vi "FPGA_ABEL_Kalman.vi"   [LabVIEW 2011]
uses:
  <vilib>/rvi/DataTransferAndStorage/Container/Common/niFpgaContainerState.ctl
  <vilib>/rvi/DataTransferAndStorage/Container/Common/niFpgaDataTypeControl.ctl
  <vilib>/rvi/DataTransferAndStorage/Container/Common/niFpgaContainerImplementationControl.ctl
  <vilib>/rvi/DataTransferAndStorage/Container/Common/niFpgaContainerArbitrationOptionsControl.ctl
  <vilib>/rvi/DataTransferAndStorage/Container/Common/niFpgaTransferTypeControl.ctl
  <vilib>/rvi/DataTransferAndStorage/Container/Common/niFpgaContainerInitializationParameters.ctl
  <vilib>/rvi/Memory/Memory_Types/niFpgaMemoryInterfaceConfiguration.ctl
  <vilib>/rvi/FIFO/Fifo_Types/niFpgaFifoControlLogicControl.ctl
  <vilib>/rvi/DataTransferAndStorage/Container/Common/niFpgaContainerMetaDataKey.ctl
  <vilib>/Platform/TimedLoop/XDataNode/timing_clust.ctl
  <vilib>/Platform/TimedLoop/XDataNode/nitl_modes.ctl
  <vilib>/Platform/TimedLoop/XDataNode/wakeup.ctl
  <vilib>/rvi/DataTransferAndStorage/Container/Common/niFpgaContainerGetUniqueNameForEmu.vi
  <vilib>/rvi/DataTransferAndStorage/Container/Common/niFpgaContainerSetEmuInfo.vi
  <vilib>/rvi/eio/common/nirviEmuReportErrorAndStop.vi
  <vilib>/rvi/FIFO/Fifo_Resource/nirvififoEmulationSetSize.vi
  Instance           3 24Saved   FPGA_ABEL_Kalman .vi
  FPGA_Global.vi
  <vilib>/rvi/interface/RandomDataEmulation/nirviRandomDataFPGAFIFO.vi
  <vilib>/rvi/interface/RandomDataEmulation/niFpgaRandomDataHandleErrors.vi
  Instance           2 24Saved   FPGA_ABEL_Kalman .vi
  <vilib>/rvi/Memory/Memory_Emulation/niFpgaMemoryEmulationValidateCache.vi
  <vilib>/rvi/Memory/Memory_Emulation/nirvimemoryEmulationManagerCache_InsertValue.vi
  <vilib>/Utility/error.llb/Clear Errors.vi
  <vilib>/rvi/Memory/Memory_Emulation/nirvimemoryEmulationManagerCache_GetValue.vi
  <vilib>/rvi/eio/common/nirviEmuTemplateMethod_errors.vi
  Instance           1 24Saved   FPGA_ABEL_Kalman .vi
  Instance           7 24Saved   FPGA_ABEL_Kalman .vi
  <vilib>/rvi/Memory/Memory_Emulation/nirvimemoryEmulationManagerCache_SetValue.vi
  <vilib>/rvi/LocalResourceManager/LocalResourceManager.xnode
  <vilib>/Platform/TimedLoop/XDataNode/XDataNode.xnode
  <vilib>/rvi/DataTransferAndStorage/Container/XNode/niFpgaContainer.xnode
  <vilib>/rvi/FIFO/Fifo_Resource/nirvififoEmulationRead.vi
  <vilib>/rvi/Arithmetic/AddSubMult/XNode/nirviSatArithmetic.xnode
  <vilib>/rvi/interface/RandomDataEmulation/nirviRandomDataFpgaReadWriteTemplate.vi
  <vilib>/eio/EIONode/EIONode.xnode
  <vilib>/rvi/Memory/Memory_Emulation/nirvimemoryEmulation.vi
  <vilib>/rvi/FIFO/Fifo_Resource/nirvififoEmulationWrite.vi
  <vilib>/Platform/TimedLoop/XDataNode/XDNodeRunTimeDep.lvlib
  <vilib>/rvi/occurrence/nirviOccurrence.lvlib
types:
  T1 = typedef "XDNodeRunTimeDep.lvlib/timing_clust.ctl" = cluster{"Expected End [f-1]":u64, "Actual End [f-1]":u64, "Finished Late? [f-1]":bool, "Expected End [i-1]":u64, "Actual End [i-1]":u64, "Finished Late? [i-1]":bool, "Expected Start [i]":u64, "Actual Start [i]":u64, "Expected Start [f]":u64, "Actual Start [f]":u64, "Source Name":string, "Structure Name":string, "Period":i64, "Deadline":i64, "Offset":i64, "Start":i64, "Priority":i32, "Timeout":i32, "Mode":T2, "Wakeup Reason":T3, "Error":errorcluster, "Source Type":string, "Secondary Source Type":string, "Global End Time":u64, "Global Start Time":u64, "Frame Duration":u64, "Iteration Duration":u64, "Assigned CPU":i32, "I/O Scan Engine Mode":u32}
  T2 = typedef "XDNodeRunTimeDep.lvlib/nitl_modes.ctl" = enum32{"No Change", "Process missed periods, maintain original phase", "Discard missed periods, maintain original phase", "Process missed periods, ignore original phase", "Discard missed periods, ignore original phase"}
  T3 = typedef "XDNodeRunTimeDep.lvlib/wakeup.ctl" = enum32{"Normal", "Aborted", "Asynchronous wakeup", "Timing source error", "Timed loop error", "Timeout"}
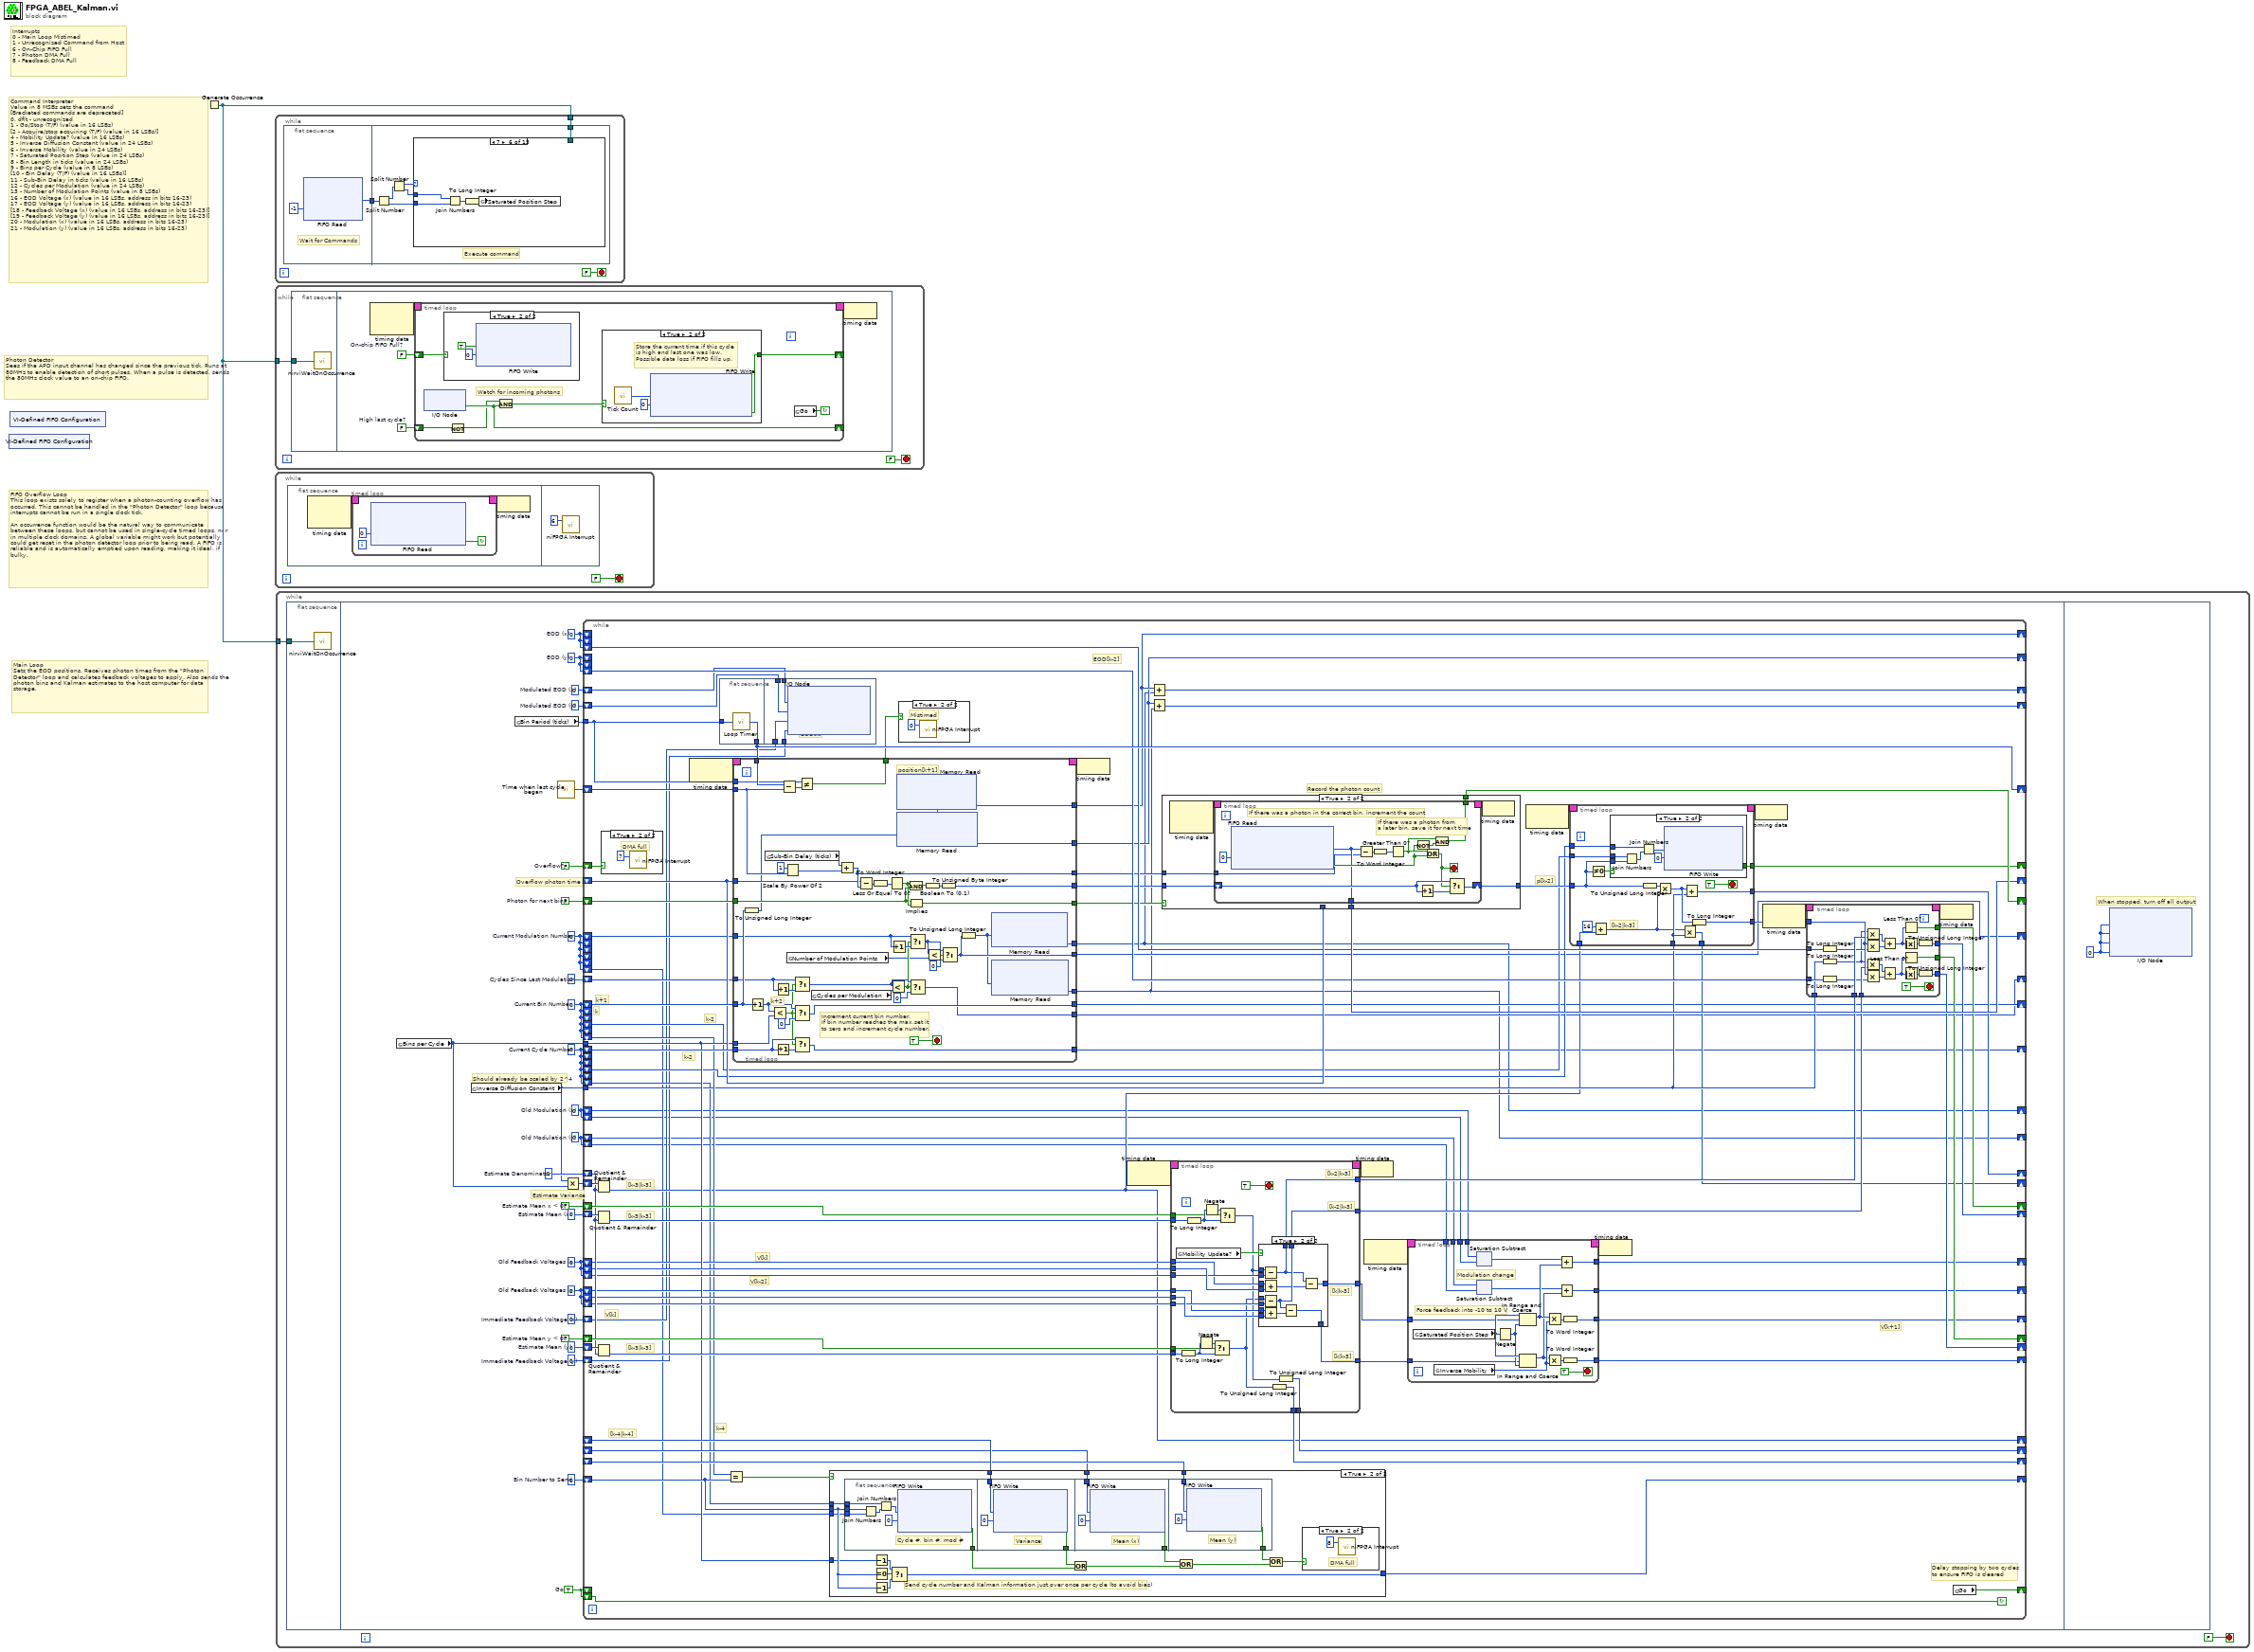
[diagram p0: block diagram]
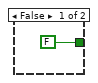
[diagram p3: hidden frame]
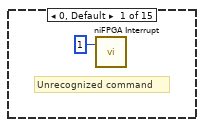
[diagram p4: hidden frame]
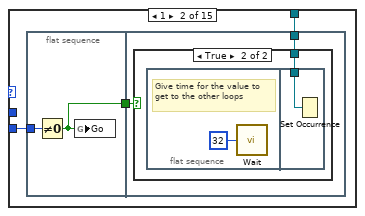
[diagram p5: hidden frame]
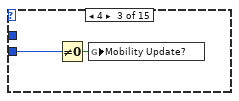
[diagram p7: hidden frame]
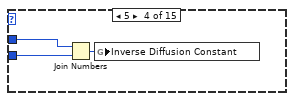
[diagram p8: hidden frame]
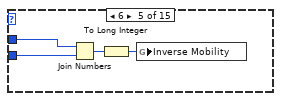
[diagram p9: hidden frame]
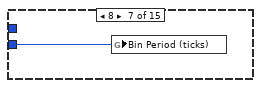
[diagram p10: hidden frame]
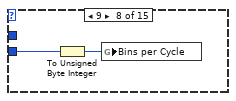
[diagram p11: hidden frame]
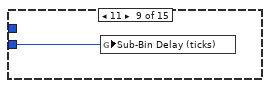
[diagram p12: hidden frame]
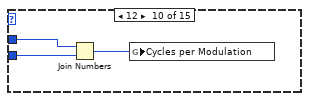
[diagram p13: hidden frame]
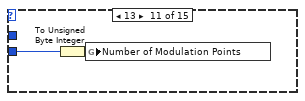
[diagram p14: hidden frame]
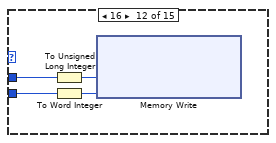
[diagram p15: hidden frame]
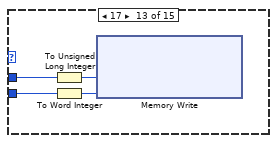
[diagram p16: hidden frame]
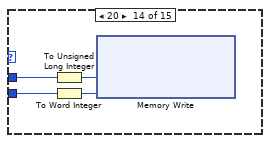
[diagram p17: hidden frame]
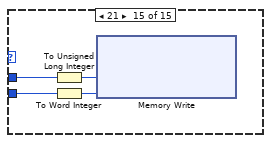
[diagram p18: hidden frame]
diagram:
  # "FIFO Overflow Loop\nThis loop exists solely to register when a photon-counting overflow has occurred. This cannot be handled in the \"Photon Detector\" loop because interrupts cannot be run in a single clock tick.\n\nAn occurrence function would be the natural way to communicate between these loops, but cannot be used in single-cycle timed loops, nor in multiple clock domains. A global variable might work but potentially could get reset in the photon detector loop prior to being read. A FIFO is reliable and is automatically emptied upon reading, making it ideal, if bulky."
  # "Interrupts\n0 - Main Loop Mistimed\n1 - Unrecognized Command from Host\n6 - On-Chip FIFO Full\n7 - Photon DMA Full\n8 - Feedback DMA Full"
  # "Command Interpreter\nValue in 8 MSBs sets the command\n[Bracketed commands are deprecated]\n0, dflt - unrecognized\n1 - Go/Stop (T/F) (value in 16 LSBs)\n[2 - Acquire/stop acquiring (T/F) (value in 16 LSBs)]\n4 - Mobility Update? (value in 16 LSBs)\n5 - Inverse Diffusion Constant (value in 24 LSBs)\n6 - Inverse Mobility (value in 24 LSBs)\n7 - Saturated Position Step (value in 24 LSBs)\n8 - Bin Length in ticks (value in 24 LSBs)\n9 - Bins per Cycle (value in 8 LSBs)\n[10 - Bin Delay (T/F) (value in 16 LSBs)]\n11 - Sub-Bin Delay in ticks (value in 16 LSBs)\n12 - Cycles per Modulation (value in 24 LSBs)\n13 - Number of Modulation Points (value in 8 LSBs)\n16 - EOD Voltage (x) (value in 16 LSBs, address in bits 16-23)\n17 - EOD Voltage (y) (value in 16 LSBs, address in bits 16-23)\n[18 - Feedback Voltage (x) (value in 16 LSBs, address in bits 16-23)]\n[19 - Feedback Voltage (y) (value in 16 LSBs, address in bits 16-23)]\n20 - Modulation (x) (value in 16 LSBs, address in bits 16-23)\n21 - Modulation (y) (value in 16 LSBs, address in bits 16-23)"
  # "Main Loop\nSets the EOD positions. Receives photon times from the \"Photon Detector\" loop and calculates feedback voltages to apply. Also sends the photon bins and Kalman estimates to the host computer for data storage."
  # "Photon Detector\nSees if the APD input channel has changed since the previous tick. Runs at 80MHz to enable detection of short pulses. When a pulse is detected, sends the 80MHz clock value to an on-chip FIFO."
  n1 = xnode "VI-Defined FIFO Configuration"() -> ()  [unwired: 1 out]
  n2 = xnode "VI-Defined FIFO Configuration"() -> ()  [unwired: 1 out]
  n3 = Generate Occurrence() -> (w1:refnum<k4>)
  n4 = while {
    tunnel: w1 -> [w2]
    stop <- FALSE stop-if-true
    n5 = flat-sequence {
      tunnel: [w5] -> w4
      tunnel: w4 -> [w12]
      tunnel: w2 -> [w7]
      frame #0 {
        # "Wait for Commands"
        n6 = xnode ("FIFO Read")("Timeout"=-1) -> ("Element"=w5:u32)  [unwired: 1 in, 2 out]
      }
      frame #1 {
        # "Execute command"
        n7 = Split Number(x=w12) -> (hi(x)=w11:u16, lo(x)=w8:u16)
        n8 = Split Number(x=w11) -> (hi(x)=w10:u8, lo(x)=w9:u8)
        n9 = case shown="7" w10 {
          tunnel: w9 -> [_ _ _ w27 w31 w35 _ _ _ w42 _ w49 w53 w57 w61]
          tunnel: w8 -> [_ w16 w25 w28 w32 w36 w37 w39 w40 w43 w45 w48 w52 w56 w60]
          tunnel: w7 -> [_ w15 _ _ _ _ _ _ _ _ _ _ _ _ _]
          frame 0, Default {
            # "Unrecognized command"
            n10 = call <vilib>:"niFPGA Interrupt.vi"("IRQ Number"=u8 1) -> ()  [unwired: 2 in]
          }
          frame 1 {
            n11 = flat-sequence {
              tunnel: w16 -> [w18]
              tunnel: [w17] -> w14
              tunnel: w15 -> [w20]
              tunnel: w14 -> [w19]
              frame #0 {
                n12 = Not Equal To 0?(x=w18) -> (x != 0?=w17:bool)
                n13 = global write "FPGA_Global.vi" "Go"(w17) -> ()
              }
              frame #1 {
                n14 = case shown="True" w19 {
                  tunnel: w20 -> [_ w21]
                  frame False {
                  }
                  frame True {
                    n15 = flat-sequence {
                      tunnel: w21 -> [w23]
                      frame #0 {
                        # "Give time for the value to get to the other loops"
                        n16 = call "Wait"("Count(Ticks)"=u8 32) -> ()  [unwired: 1 out]
                      }
                      frame #1 {
                        n17 = Set Occurrence(w23) -> ()
                      }
                    }
                  }
                }
              }
            }
          }
          frame 4 {
            n18 = Not Equal To 0?(x=w25) -> (x != 0?=w24:bool)
            n19 = global write "FPGA_Global.vi" "Mobility Update?"(w24) -> ()
          }
          frame 5 {
            n20 = Join Numbers(hi=w27, lo=w28) -> ((hi.lo)=w26:u32)
            n21 = global write "FPGA_Global.vi" "Inverse Diffusion Constant"(w26) -> ()
          }
          frame 6 {
            n22 = Join Numbers(hi=w31, lo=w32) -> ((hi.lo)=w30:u32)
            n23 = To Long Integer(number=w30) -> (32bit integer=w29:i32)
            n24 = global write "FPGA_Global.vi" "Inverse Mobility"(w29) -> ()
          }
          frame 7 {
            n25 = Join Numbers(hi=w35, lo=w36) -> ((hi.lo)=w34:u32)
            n26 = To Long Integer(number=w34) -> (32bit integer=w33:i32)
            n27 = global write "FPGA_Global.vi" "Saturated Position Step"(w33) -> ()
          }
          frame 8 {
            n28 = global write "FPGA_Global.vi" "Bin Period (ticks)"(w37) -> ()
          }
          frame 9 {
            n29 = To Unsigned Byte Integer(number=w39) -> (unsigned 8bit integer=w38:u8)
            n30 = global write "FPGA_Global.vi" "Bins per Cycle"(w38) -> ()
          }
          frame 11 {
            n31 = global write "FPGA_Global.vi" "Sub-Bin Delay (ticks)"(w40) -> ()
          }
          frame 12 {
            n32 = Join Numbers(hi=w42, lo=w43) -> ((hi.lo)=w41:u32)
            n33 = global write "FPGA_Global.vi" "Cycles per Modulation"(w41) -> ()
          }
          frame 13 {
            n34 = To Unsigned Byte Integer(number=w45) -> (unsigned 8bit integer=w44:u8)
            n35 = global write "FPGA_Global.vi" "Number of Modulation Points"(w44) -> ()
          }
          frame 16 {
            n36 = To Unsigned Long Integer(number=w49) -> (unsigned 32bit integer=w47:u32)
            n37 = To Word Integer(number=w48) -> (16bit integer=w46:i16)
            n38 = xnode ("Memory Write")("Address"=w47, "Data"=w46) -> ()  [unwired: 1 in, 1 out]
          }
          frame 17 {
            n39 = To Unsigned Long Integer(number=w53) -> (unsigned 32bit integer=w51:u32)
            n40 = To Word Integer(number=w52) -> (16bit integer=w50:i16)
            n41 = xnode ("Memory Write")("Address"=w51, "Data"=w50) -> ()  [unwired: 1 in, 1 out]
          }
          frame 20 {
            n42 = To Unsigned Long Integer(number=w57) -> (unsigned 32bit integer=w55:u32)
            n43 = To Word Integer(number=w56) -> (16bit integer=w54:i16)
            n44 = xnode ("Memory Write")("Address"=w55, "Data"=w54) -> ()  [unwired: 1 in, 1 out]
          }
          frame 21 {
            n45 = To Unsigned Long Integer(number=w61) -> (unsigned 32bit integer=w59:u32)
            n46 = To Word Integer(number=w60) -> (16bit integer=w58:i16)
            n47 = xnode ("Memory Write")("Address"=w59, "Data"=w58) -> ()  [unwired: 1 in, 1 out]
          }
        }
      }
    }
  }
  n48 = while {
    tunnel: w1 -> [w62]
    stop <- FALSE stop-if-true
    n49 = flat-sequence {
      tunnel: w62 -> [w64]
      frame #0 {
        n50 = call <vilib>:"nirviWaitOnOccurrence.vi"("occurrence"=w64) -> ()  [unwired: 4 in, 1 out]
      }
      frame #1 {
        w65 = FALSE  # On-chip FIFO Full?
        w66 = FALSE  # High last cycle?
        n51 = node-c288() -> (w68:T1)  [unwired: 2 in]
        n52 = timed-loop {
          timing: w68 -> [_]
          timing-out: [_] -> w67
          shift-right: [w71] -> _
          shift-left: w66 -> [w75]
          shift-right: [w72] -> _
          shift-left: w65 -> [w69]
          stop <- w73 continue-if-true
          # "Watch for incoming photons"
          n53 = xnode "I/O Node"() -> ("APD"=w71:bool)  [unwired: 1 in, 1 out]
          n54 = case shown="True" w69 {
            frame False {
            }
            frame True {
              n55 = xnode ("FIFO Write")("Element"=TRUE, "Timeout"=0) -> ()  [unwired: 2 in, 3 out]
            }
          }
          n56 = Not(x=w75) -> (.not. x?=w70:bool)
          n57 = And(x=w70, y=w71) -> (x .and. y?=w74:bool)
          n58 = case shown="True" w74 {
            tunnel: [FALSE ("Full") w79] -> w72
            frame False {
            }
            frame True {
              # "Store the current time if this cycle\nis high and last one was low.\nPossible data loss if FIFO fills up."
              n59 = call "Tick Count"() -> ("Tick Count(Ticks)"=w80:u16)
              n60 = xnode ("FIFO Write")("Element"=w80, "Timeout"=0) -> ("Timed Out?"=w79:bool)  [unwired: 1 in, 1 out]
            }
          }
          n61 = global read "FPGA_Global.vi" "Go"() -> (w73:bool)
        }
        n62 = node-c288(w67) -> ()
      }
    }
  }
  n63 = while {
    stop <- FALSE stop-if-true
    n64 = flat-sequence {
      frame #0 {
        n65 = node-c288() -> (w88:T1)  [unwired: 2 in]
        n66 = timed-loop {
          timing: w88 -> [_]
          timing-out: [_] -> w87
          stop <- w89 continue-if-true
          n67 = xnode ("FIFO Read")("Timeout"=0) -> ("Timed Out?"=w89:bool)  [unwired: 1 in, 2 out]
        }
        n68 = node-c288(w87) -> ()
      }
      frame #1 {
        n69 = call <vilib>:"niFPGA Interrupt.vi"("IRQ Number"=u8 6) -> ()  [unwired: 2 in]
      }
    }
  }
  n70 = while {
    tunnel: w1 -> [w96]
    stop <- FALSE stop-if-true
    n71 = flat-sequence {
      tunnel: w96 -> [w98]
      frame #0 {
        n72 = call <vilib>:"nirviWaitOnOccurrence.vi"("occurrence"=w98) -> ()  [unwired: 4 in, 1 out]
      }
      frame #1 {
        w100 = i16 0  # Old Modulation (y)
        w99 = i16 0  # Old Modulation (x)
        w102 = i16 0  # Modulated EOD (y)
        w103 = i16 0  # Modulated EOD (x)
        w101 = u8 0  # Current Modulation Number
        w104 = u32 0  # Cycles Since Last Modulation
        w110 = u8 0  # Bin Number to Send
        w111 = TRUE  # Go
        w108 = 0  # Old Feedback Voltages (y)
        w109 = 0  # Old Feedback Voltages (x)
        w112 = i16 0  # Immediate Feedback Voltage (y)
        w113 = i16 0  # Immediate Feedback Voltage (x)
        w118 = u32 1  # Estimate Denominator
        w120 = FALSE  # Estimate Mean y < 0?
        w121 = FALSE  # Estimate Mean x < 0?
        w122 = u32 0  # Estimate Mean (y)
        w123 = u32 0  # Estimate Mean (x)
        w124 = FALSE  # Overflow?
        w125 = FALSE  # Photon for next bin?
        w114 = i16 0  # EOD (y)
        w115 = i16 0  # EOD (x)
        w106 = u16 0  # Current Cycle Number
        w107 = u8 0  # Current Bin Number
        # "Should already be scaled by 2^4"
        # "Estimate Variance"
        # "Overflow photon time"
        n73 = global read "FPGA_Global.vi" "Bins per Cycle"() -> (w116:u8)
        n74 = global read "FPGA_Global.vi" "Inverse Diffusion Constant"() -> (w105:u32)
        n75 = global read "FPGA_Global.vi" "Bin Period (ticks)"() -> (w119:u16)
        n76 = call "Time when last cycle began"() -> ("Tick Count(Ticks)"=w126:u16)
        n77 = Multiply(x=w105, y=w116) -> (x*y=w117:u32)
        n78 = while {
          tunnel: w119 -> [w215]
          shift-right: [w139] -> _
          shift-left: w115 -> [_]
          shift-right: [w138] -> _
          shift-left: w114 -> [_]
          shift-right: [w147] -> _
          shift-left: w107 -> [w219]
          tunnel: w116 -> [w163]
          shift-right: [w148] -> _
          shift-left: w106 -> [w218]
          shift-left: w114 -> [_]
          shift-left: w115 -> [_]
          shift-right: [w216] -> _
          shift-left: w126 -> [w217]
          shift-right: [w214] -> _
          shift-left: w125 -> [w213]
          shift-right: [w212] -> _
          shift-left: _ -> [w211]
          shift-left: w106 -> [_]
          shift-left: w106 -> [_]
          shift-left: w107 -> [_]
          shift-left: w107 -> [_]
          shift-right: [w207] -> _
          shift-left: w124 -> [w206]
          shift-right: [w187] -> _
          shift-left: w123 -> [w200]
          shift-right: [w153] -> _
          shift-left: w117 -> [w201]
          tunnel: w105 -> [w156]
          shift-right: [w189] -> _
          shift-left: w122 -> [w198]
          shift-right: [w170] -> _
          shift-left: w113 -> [w141]
          shift-right: [w169] -> _
          shift-left: w112 -> [w140]
          shift-right: [w188] -> _
          shift-left: w120 -> [w202]
          shift-right: [w186] -> _
          shift-left: w121 -> [w203]
          shift-right: [w196] -> _
          shift-left: w118 -> [w181]
          shift-right: [w154] -> _
          shift-left: _ -> [w182]
          shift-right: [w195] -> _
          shift-left: _ -> [w179]
          shift-right: [w194] -> _
          shift-left: _ -> [w180]
          shift-left: w115 -> [w177]
          shift-left: w114 -> [w178]
          shift-right: [w167] -> _
          shift-left: w109 -> [w175]
          shift-left: w109 -> [w176]
          shift-right: [w168] -> _
          shift-left: w108 -> [w173]
          shift-left: w108 -> [w174]
          shift-right: [w166] -> _
          shift-left: w111 -> [_]
          shift-left: w111 -> [w165]
          shift-right: [w162] -> _
          shift-left: w110 -> [w164]
          shift-left: w107 -> [w161]
          shift-left: w107 -> [_]
          shift-left: w106 -> [w160]
          shift-left: w106 -> [_]
          shift-left: w109 -> [w159]
          shift-left: w108 -> [w158]
          shift-left: w107 -> [w157]
          shift-left: w106 -> [w155]
          shift-right: [w142] -> _
          shift-left: w104 -> [w150]
          shift-right: [w143] -> _
          shift-left: w101 -> [w149]
          shift-right: [w135] -> _
          shift-left: w103 -> [w137]
          shift-right: [w134] -> _
          shift-left: w102 -> [w136]
          shift-left: w101 -> [_]
          shift-left: w101 -> [_]
          shift-left: w101 -> [_]
          shift-left: w101 -> [_]
          shift-left: w101 -> [w133]
          shift-right: [w130] -> _
          shift-left: w99 -> [w131]
          shift-right: [w129] -> _
          shift-left: w100 -> [w128]
          shift-left: w99 -> [w132]
          shift-left: w100 -> [w127]
          stop <- w165 continue-if-true
          # "V[k-2]"
          # "V[k]"
          # "EOD[k-2]"
          # "k-2"
          # "k-4"
          # "Delay stopping by two cycles\nto ensure FIFO is cleared"
          # "V[k]"
          # "[k-3|k-3]"
          # "[k-3|k-3]"
          # "[k-4|k-4]"
          # "[k-3|k-3]"
          # "k-2"
          # "k"
          # "k+1"
          # "p[k-2]"
          # "V[k+1]"
          # "Record the photon count"
          n79 = Quotient & Remainder(x=w201, y=w181) -> (floor(x/y)=w154:u32)  [unwired: 1 out]
          n80 = Quotient & Remainder(x=w200, y=w181) -> (floor(x/y)=w199:u32)  [unwired: 1 out]
          n81 = Quotient & Remainder(x=w198, y=w181) -> (floor(x/y)=w197:u32)  [unwired: 1 out]
          n82 = case shown="True" w206 {
            frame False {
            }
            frame True {
              # "DMA full"
              n83 = call <vilib>:"niFPGA Interrupt.vi"("IRQ Number"=u8 7) -> ()  [unwired: 2 in]
            }
          }
          n84 = node-c288() -> (w221:T1)  [unwired: 1 in]
          n85 = flat-sequence {
            tunnel: w215 -> [w497]
            tunnel: [w496] -> w216
            tunnel: w141 -> [w501]
            tunnel: w140 -> [w500]
            tunnel: w137 -> [w499]
            tunnel: w136 -> [w498]
            frame #0 {
              n86 = call "Loop Timer"("Count(Ticks)"=w497) -> ("Tick Count(Ticks)"=w496:u16)
            }
            frame #1 {
              # "EOD[k]"
              n87 = xnode ("I/O Node")("EODDriver(x)"=w499, "EODDriver(y)"=w498, "FeedbackVoltage (x)"=w501, "FeedbackVoltage(y)"=w500) -> ()  [unwired: 4 in, 4 out]
            }
          }
          n88 = Equal?(x=w157, y=w164) -> (x = y?=w193:bool)
          n89 = timed-loop {
            timing: w221 -> [_]
            timing-out: [_] -> w220
            tunnel: w219 -> [w487]
            tunnel: [w490] -> w139
            tunnel: [w489] -> w138
            tunnel: w163 -> [w486]
            tunnel: [w485] -> w147
            tunnel: w218 -> [w482]
            tunnel: [w481] -> w148
            tunnel: w216 -> [w480]
            tunnel: w217 -> [w477]
            tunnel: w215 -> [w478]
            tunnel: [w466] -> w146
            tunnel: w213 -> [w469]
            tunnel: [w468] -> w145
            tunnel: [w467] -> w144
            tunnel: w211 -> [w465]
            tunnel: [w464] -> w210
            tunnel: w150 -> [w459]
            tunnel: w149 -> [w455]
            tunnel: [w450] -> w143
            tunnel: [w448] -> w142
            tunnel: [w447] -> w130
            tunnel: [w446] -> w129
            stop <- TRUE stop-if-true
            # "k+2"
            # "position[k+1]"
            # "Increment current bin number.\nIf bin number reaches the max,set it\nto zero and increment cycle number."
            n90 = To Unsigned Long Integer(number=w487) -> (unsigned 32bit integer=w463:u32)
            n91 = Increment(x=w487) -> (x+1=w488:u8)
            n92 = global read "FPGA_Global.vi" "Sub-Bin Delay (ticks)"() -> (w462:u16)
            n93 = Less?(x=w488, y=w486) -> (x < y?=w460:bool)
            n94 = Increment(x=w459) -> (x+1=w461:u32)
            n95 = Increment(x=w482) -> (x+1=w483:u16)
            n96 = Subtract(x=w480, y=w477) -> (x-y=w479:u16)
            n97 = Scale By Power Of 2(n=1, x=w477) -> (x*2^n=w475:u16)
            n98 = global read "FPGA_Global.vi" "Number of Modulation Points"() -> (w445:u8)
            n99 = Select(t=w459, s=w460, f=w461) -> (s? t:f=w458:u32)
            n100 = Select(t=w488, s=w460, f=u8 0 ("Current Bin Number")) -> (s? t:f=w485:u8)
            n101 = Select(t=w482, s=w460, f=w483) -> (s? t:f=w481:u16)
            n102 = Not Equal?(x=w478, y=w479) -> (x != y?=w464:bool)
            n103 = global read "FPGA_Global.vi" "Cycles per Modulation"() -> (w444:u32)
            n104 = Add(x=w462, y=w475) -> (x+y=w466:u16)
            n105 = Subtract(x=w465, y=w466) -> (x-y=w471:u16)
            n106 = To Word Integer(number=w471) -> (16bit integer=w472:i16)
            n107 = Less Or Equal To 0?(x=w472) -> (x <= 0?=w470:bool)
            n108 = Less?(x=w458, y=w444) -> (x < y?=w454:bool)
            n109 = Increment(x=w455) -> (x+1=w456:u8)
            n110 = xnode ("Memory Read")("Address"=w463) -> ("Data"=w490:i16)  [unwired: 1 in, 1 out]
            n111 = xnode ("Memory Read")("Address"=w463) -> ("Data"=w489:i16)  [unwired: 1 in, 1 out]
            n112 = And(x=w470, y=w469) -> (x .and. y?=w474:bool)
            n113 = Implies(1:w470, 2:w469) -> (0:w467:bool)
            n114 = Select(t=w455, s=w454, f=w456) -> (s? t:f=w451:u8)
            n115 = Select(t=w458, s=w454, f=u32 0) -> (s? t:f=w448:u32)
            n116 = Boolean To (0,1)(Boolean=w474) -> (0, 1=w473:i16)
            n117 = Less?(x=w451, y=w445) -> (x < y?=w453:bool)
            n118 = To Unsigned Byte Integer(number=w473) -> (unsigned 8bit integer=w468:u8)
            n119 = Select(t=w451, s=w453, f=u8 0) -> (s? t:f=w450:u8)
            n120 = To Unsigned Long Integer(number=w450) -> (unsigned 32bit integer=w449:u32)
            n121 = xnode ("Memory Read")("Address"=w449) -> ("Data"=w447:i16)  [unwired: 1 in, 1 out]
            n122 = xnode ("Memory Read")("Address"=w449) -> ("Data"=w446:i16)  [unwired: 1 in, 1 out]
          }
          n123 = case shown="True" w193 {
            tunnel: w179 -> [_ w326]
            tunnel: w182 -> [_ w325]
            tunnel: w155 -> [_ w324]
            tunnel: w180 -> [_ w320]
            tunnel: w164 -> [w308 w315]
            tunnel: w163 -> [_ w311]
            tunnel: [w308 w312] -> w162
            tunnel: w133 -> [_ w309]
            frame False {
            }
            frame True {
              # "Send cycle number and Kalman information just over once per cycle (to avoid bias)"
              n124 = flat-sequence {
                tunnel: w324 -> [w332]
                tunnel: [w333] -> w323
                tunnel: w315 -> [w329]
                tunnel: w309 -> [w328]
                tunnel: [w335] -> w322
                tunnel: w325 -> [w336]
                tunnel: w326 -> [w339]
                tunnel: [w338] -> w321
                tunnel: [w341] -> w318
                tunnel: w320 -> [w342]
                frame #0 {
                  # "Cycle #, bin #, mod #"
                  n125 = Join Numbers(hi=w329, lo=w328) -> ((hi.lo)=w330:u16)
                  n126 = Join Numbers(hi=w332, lo=w330) -> ((hi.lo)=w331:u32)
                  n127 = xnode ("FIFO Write")("Element"=w331, "Timeout"=0) -> ("Timed Out?"=w333:bool)  [unwired: 1 in, 1 out]
                }
                frame #1 {
                  # "Variance"
                  n128 = xnode ("FIFO Write")("Element"=w336, "Timeout"=0) -> ("Timed Out?"=w335:bool)  [unwired: 1 in, 1 out]
                }
                frame #2 {
                  # "Mean (x)"
                  n129 = xnode ("FIFO Write")("Element"=w339, "Timeout"=0) -> ("Timed Out?"=w338:bool)  [unwired: 1 in, 1 out]
                }
                frame #3 {
                  # "Mean (y)"
                  n130 = xnode ("FIFO Write")("Element"=w342, "Timeout"=0) -> ("Timed Out?"=w341:bool)  [unwired: 1 in, 1 out]
                }
              }
              n131 = Decrement(x=w311) -> (x-1=w310:u8)
              n132 = Equal To 0?(x=w315) -> (x = 0?=w314:bool)
              n133 = Decrement(x=w315) -> (x-1=w313:u8)
              n134 = Select(t=w310, s=w314, f=w313) -> (s? t:f=w312:u8)
              n135 = Or(x=w322, y=w323) -> (x .or. y?=w317:bool)
              n136 = Or(x=w321, y=w317) -> (x .or. y?=w319:bool)
              n137 = Or(x=w318, y=w319) -> (x .or. y?=w316:bool)
              n138 = case shown="True" w316 {
                frame False {
                }
                frame True {
                  # "DMA full"
                  n139 = call <vilib>:"niFPGA Interrupt.vi"("IRQ Number"=u8 8) -> ()  [unwired: 2 in]
                }
              }
            }
          }
          n140 = case shown="True" w210 {
            frame False {
            }
            frame True {
              # "Mistimed"
              n141 = call <vilib>:"niFPGA Interrupt.vi"("IRQ Number"=u8 0) -> ()  [unwired: 2 in]
            }
          }
          n142 = node-c288(w220) -> ()
          n143 = node-c288() -> (w205:T1)  [unwired: 1 in]
          n144 = Add(x=w139, y=w130) -> (x+y=w135:i16)
          n145 = Add(x=w138, y=w129) -> (x+y=w134:i16)
          n146 = case shown="True" w144 {
            tunnel: w146 -> [_ w424]
            tunnel: [u8 0 w423] -> w192
            tunnel: [TRUE w422] -> w214
            tunnel: w145 -> [_ w421]
            tunnel: [w418 w420] -> w212
            tunnel: w211 -> [w418 _]
            frame False {
              # "Still not time to use the photon from last cycle!"
            }
            frame True {
              n147 = node-c288() -> (w426:T1)  [unwired: 2 in]
              n148 = timed-loop {
                timing: w426 -> [_]
                timing-out: [_] -> w425
                tunnel: w424 -> [w429]
                shift-right: [w438] -> w423
                shift-left: w421 -> [w436]
                tunnel: [w433] -> w422
                tunnel: [w430] -> w420
                stop <- w435 stop-if-true
                # "If there was a photon in the correct bin, increment the count"
                # "If there was a photon from\na later bin, save it for next time"
                n149 = xnode ("FIFO Read")("Timeout"=0) -> ("Element"=w430:u16, "Timed Out?"=w432:bool)  [unwired: 1 in, 1 out]
                n150 = Subtract(x=w430, y=w429) -> (x-y=w428:u16)
                n151 = To Word Integer(number=w428) -> (16bit integer=w427:i16)
                n152 = Greater Than 0?(x=w427) -> (x > 0?=w434:bool)
                n153 = Not(x=w432) -> (.not. x?=w431:bool)
                n154 = Increment(x=w436) -> (x+1=w437:u8)
                n155 = Or(x=w434, y=w432) -> (x .or. y?=w435:bool)
                n156 = And(x=w434, y=w431) -> (x .and. y?=w433:bool)
                n157 = Select(t=w436, s=w435, f=w437) -> (s? t:f=w438:u8)
              }
              n158 = node-c288(w425) -> ()
            }
          }
          n159 = timed-loop {
            timing: w205 -> [_]
            timing-out: [_] -> w204
            tunnel: w197 -> [w366]
            tunnel: w199 -> [w365]
            tunnel: [w346] -> w184
            tunnel: [w347] -> w183
            tunnel: w176 -> [w352]
            tunnel: w174 -> [w350]
            tunnel: w203 -> [w362]
            tunnel: w202 -> [w359]
            tunnel: [w358] -> w195
            tunnel: [w357] -> w194
            tunnel: w173 -> [w351]
            tunnel: [w356] -> w151
            tunnel: w175 -> [w353]
            tunnel: [w355] -> w152
            tunnel: w159 -> [w349]
            tunnel: w158 -> [w348]
            stop <- TRUE stop-if-true
            # "[k-2|k-3]"
            # "[k|k-3]"
            # "[k|k-3]"
            # "[k-2|k-3]"
            n160 = global read "FPGA_Global.vi" "Mobility Update?"() -> (w354:bool)
            n161 = To Long Integer(number=w366) -> (32bit integer=w360:i32)
            n162 = To Long Integer(number=w365) -> (32bit integer=w363:i32)
            n163 = Negate(x=w360) -> (-x=w361:i32)
            n164 = Negate(x=w363) -> (-x=w364:i32)
            n165 = Select(t=w361, s=w359, f=w360) -> (s? t:f=w344:i32)
            n166 = Select(t=w364, s=w362, f=w363) -> (s? t:f=w345:i32)
            n167 = case shown="True" w354 {
              tunnel: w350 -> [_ w383]
              tunnel: w352 -> [_ w382]
              tunnel: w345 -> [w369 w381]
              tunnel: w344 -> [w368 w380]
              tunnel: w351 -> [_ w371]
              tunnel: [w368 w379] -> w347
              tunnel: [w368 w378] -> w356
              tunnel: w353 -> [_ w375]
              tunnel: [w369 w377] -> w346
              tunnel: [w369 w376] -> w355
              tunnel: w349 -> [_ w374]
              tunnel: w348 -> [_ w370]
              frame False {
              }
              frame True {
                n168 = Subtract(x=w381, y=w382) -> (x-y=w377:i32)
                n169 = Add(x=w374, y=w375) -> (x+y=w373:i32)
                n170 = Subtract(x=w380, y=w383) -> (x-y=w379:i32)
                n171 = Add(x=w370, y=w371) -> (x+y=w372:i32)
                n172 = Subtract(x=w379, y=w372) -> (x-y=w378:i32)
                n173 = Subtract(x=w377, y=w373) -> (x-y=w376:i32)
              }
            }
            n174 = To Unsigned Long Integer(number=w344) -> (unsigned 32bit integer=w357:u32)
            n175 = To Unsigned Long Integer(number=w345) -> (unsigned 32bit integer=w358:u32)
          }
          n176 = node-c288(w204) -> ()
          n177 = node-c288() -> (w172:T1)  [unwired: 1 in]
          n178 = timed-loop {
            timing: w172 -> [_]
            timing-out: [_] -> w171
            tunnel: [w236] -> w170
            tunnel: [w235] -> w169
            tunnel: [w224] -> w168
            tunnel: [w228] -> w167
            tunnel: w151 -> [w234]
            tunnel: w152 -> [w233]
            tunnel: w132 -> [w231]
            tunnel: w131 -> [w230]
            tunnel: w128 -> [w226]
            tunnel: w127 -> [w225]
            stop <- TRUE stop-if-true
            # "Modulation change"
            # "Force feedback into -10 to 10 V"
            n179 = global read "FPGA_Global.vi" "Saturated Position Step"() -> (w238:i32)
            n180 = global read "FPGA_Global.vi" "Inverse Mobility"() -> (w240:i32)
            n181 = xnode "Saturation Subtract"("x"=w230, "y"=w231) -> ("x-y"=w222:i32)
            n182 = xnode "Saturation Subtract"("x"=w226, "y"=w225) -> ("x-y"=w223:i32)
            n183 = Negate(x=w238) -> (-x=w237:i32)
            n184 = In Range and Coerce(upper limit=w238, x=w233, lower limit=w237) -> (coerced(x)=w229:i32)  [unwired: 1 out]
            n185 = In Range and Coerce(upper limit=w238, x=w234, lower limit=w237) -> (coerced(x)=w227:i32)  [unwired: 1 out]
            n186 = Multiply(x=w229, y=w240) -> (x*y=w239:i32)
            n187 = Multiply(x=w227, y=w240) -> (x*y=w241:i32)
            n188 = Add(x=w222, y=w229) -> (x+y=w228:i32)
            n189 = Add(x=w223, y=w227) -> (x+y=w224:i32)
            n190 = To Word Integer(number=w239) -> (16bit integer=w236:i16)
            n191 = To Word Integer(number=w241) -> (16bit integer=w235:i16)
          }
          n192 = node-c288() -> (w209:T1)  [unwired: 1 in]
          n193 = timed-loop {
            timing: w209 -> [_]
            timing-out: [_] -> w208
            tunnel: w192 -> [w397]
            tunnel: w160 -> [w401]
            tunnel: w161 -> [w400]
            tunnel: [w399] -> w207
            tunnel: w156 -> [w393]
            tunnel: [w394] -> w196
            tunnel: [w395] -> w185
            tunnel: w154 -> [w391]
            tunnel: [w392] -> w153
            stop <- TRUE stop-if-true
            # "[k-2|k-3]"
            n194 = Not Equal To 0?(x=w397) -> (x != 0?=w402:bool)
            n195 = Add(x=u32 16, y=w391) -> (x+y=w390:u32)
            n196 = case shown="True" w402 {
              tunnel: w397 -> [_ w410]
              tunnel: w401 -> [_ w409]
              tunnel: w400 -> [_ w408]
              tunnel: [FALSE ("Full") w405] -> w399
              frame False {
              }
              frame True {
                n197 = Join Numbers(hi=w408, lo=w410) -> ((hi.lo)=w411:u16)
                n198 = Join Numbers(hi=w409, lo=w411) -> ((hi.lo)=w407:u32)
                n199 = xnode ("FIFO Write")("Element"=w407, "Timeout"=0) -> ("Timed Out?"=w405:bool)  [unwired: 1 in, 1 out]
              }
            }
            n200 = To Unsigned Long Integer(number=w397) -> (unsigned 32bit integer=w398:u32)
            n201 = Multiply(x=w398, y=w390) -> (x*y=w396:u32)
            n202 = Multiply(x=w390, y=w393) -> (x*y=w392:u32)
            n203 = Add(x=w396, y=w393) -> (x+y=w394:u32)
            n204 = To Long Integer(number=w396) -> (32bit integer=w395:i32)
          }
          n205 = node-c288(w171) -> ()
          n206 = node-c288(w208) -> ()
          n207 = node-c288() -> (w191:T1)  [unwired: 1 in]
          n208 = timed-loop {
            timing: w191 -> [_]
            timing-out: [_] -> w190
            tunnel: [w299] -> w189
            tunnel: [w298] -> w188
            tunnel: [w297] -> w187
            tunnel: [w296] -> w186
            tunnel: w185 -> [w293]
            tunnel: w177 -> [w287]
            tunnel: w178 -> [w284]
            tunnel: w156 -> [w283]
            tunnel: w184 -> [w290]
            tunnel: w183 -> [w289]
            stop <- TRUE stop-if-true
            n209 = To Long Integer(number=w287) -> (32bit integer=w286:i32)
            n210 = To Long Integer(number=w283) -> (32bit integer=w282:i32)
            n211 = To Long Integer(number=w284) -> (32bit integer=w285:i32)
            n212 = Multiply(x=w282, y=w290) -> (x*y=w292:i32)
            n213 = Multiply(x=w293, y=w286) -> (x*y=w295:i32)
            n214 = Multiply(x=w282, y=w289) -> (x*y=w291:i32)
            n215 = Multiply(x=w293, y=w285) -> (x*y=w294:i32)
            n216 = Add(x=w292, y=w295) -> (x+y=w302:i32)
            n217 = Add(x=w291, y=w294) -> (x+y=w300:i32)
            n218 = Less Than 0?(x=w302) -> (x < 0?=w296:bool)
            n219 = Absolute Value(x=w302) -> (abs(x)=w303:i32)
            n220 = Less Than 0?(x=w300) -> (x < 0?=w298:bool)
            n221 = Absolute Value(x=w300) -> (abs(x)=w301:i32)
            n222 = To Unsigned Long Integer(number=w303) -> (unsigned 32bit integer=w297:u32)
            n223 = To Unsigned Long Integer(number=w301) -> (unsigned 32bit integer=w299:u32)
          }
          n224 = node-c288(w190) -> ()
          n225 = global read "FPGA_Global.vi" "Go"() -> (w166:bool)
        }
      }
      frame #2 {
        w502 = i16 0 ("Feedback Voltage (y)")
        # "When stopped, turn off all output"
        n226 = xnode "I/O Node"("EODDriver(x)"=w502, "EODDriver(y)"=w502, "FeedbackVoltage (x)"=w502, "FeedbackVoltage(y)"=w502) -> ()  [unwired: 4 in, 4 out]
      }
    }
  }
